vi "ParseXMLParams.vi"(0 "Parameter String":string) -> (1 "Names":string[](array[string]), 2 "Values":string[](array[string]))   [LabVIEW 2020]
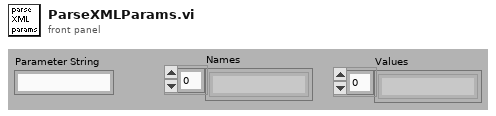
[diagram p1: front panel]
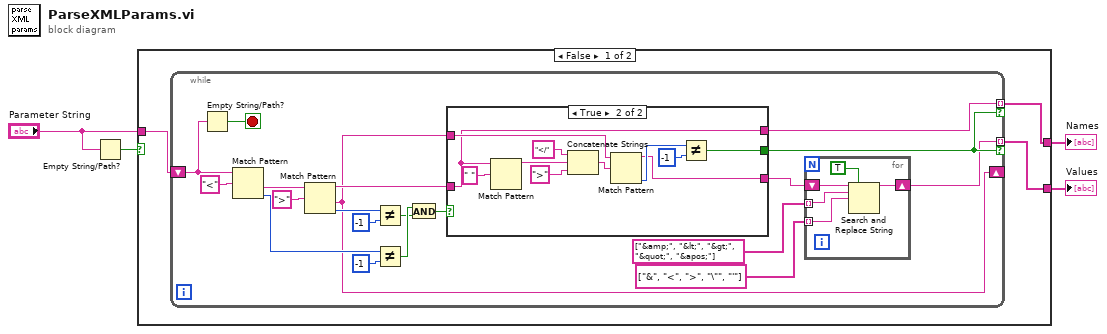
[diagram p0: block diagram]
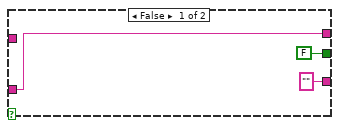
[diagram p2: hidden frame]
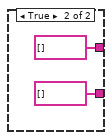
[diagram p3: hidden frame]
diagram:
  n1 = Empty String/Path?(string/path="Parameter String") -> (empty?=w2:bool)
  n2 = case shown="False" w2 {
    tunnel: "Parameter String" -> [w7 _]
    tunnel: [w5 string[] []] -> w4
    tunnel: [w6 string[] []] -> w3
    frame False {
      n3 = while {
        tunnel: [w10] -> w5 mode=indexing if=w13
        shift-right: [w11] -> _
        shift-left: w7 -> [w16]
        tunnel: [w14] -> w6 mode=indexing if=w13
        stop <- w15 stop-if-true
        n4 = Empty String/Path?(string/path=w16) -> (empty?=w15:bool)
        n5 = Match Pattern(string=w16, regular expression="<") -> (after substring=w26:string, offset past match=w24:i32)  [unwired: 1 in, 2 out]
        n6 = Match Pattern(string=w26, regular expression=">") -> (before substring=w18:string, after substring=w11:string, offset past match=w17:i32)  [unwired: 1 in, 1 out]
        n7 = Not Equal?(x=w17, y=-1) -> (x != y?=w20:bool)
        n8 = Not Equal?(x=w24, y=-1) -> (x != y?=w21:bool)
        n9 = And(x=w21, y=w20) -> (x .and. y?=w19:bool)
        n10 = case shown="True" w19 {
          tunnel: w18 -> [w35 w38]
          tunnel: [w35 w38] -> w14
          tunnel: w11 -> [_ w40]
          tunnel: ["" ("Parameter String") w36] -> w12
          tunnel: [FALSE w39] -> w13
          frame False {
          }
          frame True {
            n11 = Match Pattern(string=w38, regular expression=" ") -> (before substring=w44:string)  [unwired: 1 in, 3 out]
            n12 = Concatenate Strings("</" ("string"), w44, ">" ("string")) -> (w42:string)
            n13 = Match Pattern(string=w40, regular expression=w42) -> (before substring=w36:string, offset past match=w37:i32)  [unwired: 1 in, 2 out]
            n14 = Not Equal?(x=w37, y=-1) -> (x != y?=w39:bool)
          }
        }
        n15 = for {
          shift-right: [w30] -> w10
          shift-left: w12 -> [w31]
          tunnel: string[] ["&amp;", "&lt;", "&gt;", "&quot;", "&apos;"] -> [w29] mode=indexing
          tunnel: string[] ["&", "<", ">", "\"", "'"] -> [w28] mode=indexing
          n16 = Search and Replace String(replace all?=TRUE ("replace all? (F)"), input string=w31, search string=w29, replace string=w28) -> (result string=w30:string)  [unwired: 4 in, 3 out]
        }
      }
    }
    frame True {
    }
  }
  "Values" <- w4
  "Names" <- w3
